vi "NapovedaACC(subVI).vi"() -> ()   [LabVIEW 2026]
panel:
  in  "Close":bool
  # "1. Vybalte a připevněte akcelerometr na sledované místo nebo nechte ležet na stole (záleží na úloze) \n2. Do bílé propojky k nápisu ACC zapojte propojovací kabel a jeho druhý konec do portu A3.\n3. Zapněte PLUX BITalino (LED musí pulsovat).\n4. Spusťte měření."
  # "Zapojení akcelerometru"
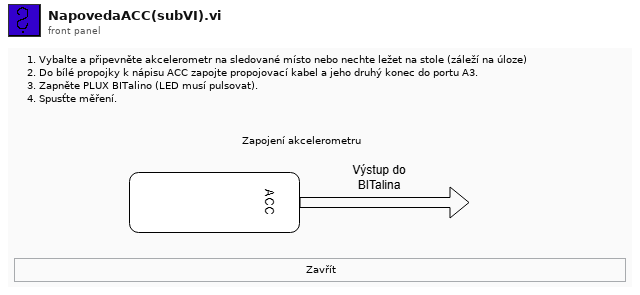
[diagram p1: front panel]
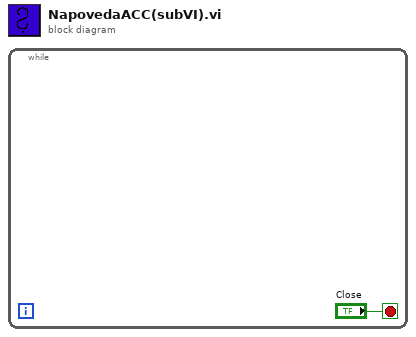
[diagram p0: block diagram]
diagram:
  n1 = while {
    stop <- "Close" stop-if-true
  }
